vi "read command.vi"(8 "error in (no error)":errorcluster, 11 "File interpreter in":refnum<class "File interpreter.lvclass">) -> (0 "error out":errorcluster, 2 "command":string, 3 "File interpreter out":refnum<class "File interpreter.lvclass">)   [LabVIEW 2018, in "File interpreter.lvclass"]
uses:
  File interpreter.lvclass
  File interpreter.lvclass/File interpreter.ctl
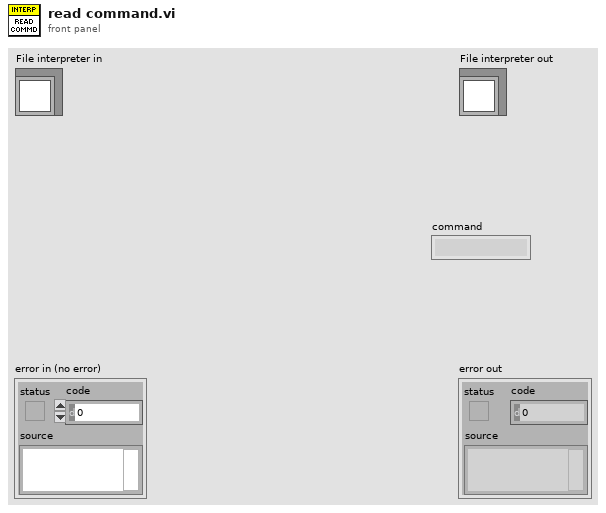
[diagram p1: front panel]
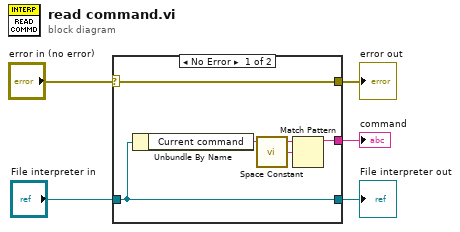
[diagram p0: block diagram]
diagram:
  n1 = case shown="No Error" "error in (no error)" {
    selector: "error in (no error)" -> [w10 w12]
    tunnel: [w10 w12] -> w4
    tunnel: [w9 w11] -> w2
    tunnel: "File interpreter in" -> [w9 w11]
    tunnel: [w6 _] -> w1
    frame No Error {
      n2 = Unbundle By Name(w9) -> ("Current command"=w7:string)
      n3 = call <vilib>:"Space Constant.vi"() -> ("String"=w8:string)
      n4 = Match Pattern(string=w7, regular expression=w8) -> (before substring=w6:string)  [unwired: 1 in, 3 out]
    }
    frame Error {
    }
  }
  "error out" <- w4
  "File interpreter out" <- w2
  "command" <- w1
